vi "Begin.vi"(8 "error in":errorcluster) -> (0 "error out":errorcluster)   [LabVIEW 2015]
doc: "Called before other user functions, this VI is expected to open initial I/O refnums, load in file data, and do all program initialization. Notice that the <B>error out</B> terminal is simply used for data flow. Wiring it to other structures or subVIs ensures that this VI runs first."
uses:
  <vilib>/Rock Robotics/WPI/DriverStation/WPI_DriverStationRobotMode2.ctl
  <vilib>/Rock Robotics/WPI/Joystick/WPI_JoystickDeviceEnum.ctl
  <vilib>/Rock Robotics/SystemInterfaces/spilib/spi_bus.ctl
  <vilib>/Rock Robotics/WPI/SafetyOutput/WPI_SafetyOutputConfigMenu.ctl
  <vilib>/Rock Robotics/SystemInterfaces/DIO/FPGA_DIOPWMChannel.ctl
  <vilib>/Rock Robotics/SystemInterfaces/DIO/FPGA_DIOChannel.ctl
  <vilib>/Rock Robotics/WPI/Encoder/WPI_EncoderType.ctl
  <vilib>/Rock Robotics/WPI/CAN/TalonSRX/WPI_CANTalonSRX_APIControlMode.ctl
  Robot Global Data.vi
  <vilib>/Rock Robotics/Network Tables/NT Write String Array.vi
  <vilib>/Rock Robotics/WPI/Gyro/WPI_GyroXRS450_SPI_Open.vi
  GyroPlaceHolder.vi
  GyroLastValue.vi
  <vilib>/Rock Robotics/WPI/RobotDrive/WPI_RobotDriveOpen4MotorWithCANTalonSRX.vi
  <vilib>/Rock Robotics/WPI/MotorControl/WPI_MotorControlOpen TalonSRX.vi
  <vilib>/Rock Robotics/WPI/Counter/WPI_CounterDigitalInputToDigitalSource.vi
  <vilib>/Rock Robotics/WPI/MotorControl/WPI_MotorControlOpenCANTalonSRX.vi
  <vilib>/Rock Robotics/WPI/Switch/WPI_SwitchOpenLimit.vi
  <vilib>/Rock Robotics/WPI/Accelerometer/InternalAccelerometer/WPI_AccelerometerInternalOpen.vi
  <vilib>/Rock Robotics/SystemInterfaces/AI/FPGA_AIGyroChannel.ctl
  <vilib>/Rock Robotics/WPI/MotorControl/WPI_MotorControlOpen Talon.vi
  <vilib>/Rock Robotics/WPI/Gyro/WPI_GyroAnalogOpen.vi
  <vilib>/Rock Robotics/SystemInterfaces/i2clib/i2c_bus.ctl
  <vilib>/Rock Robotics/WPI/Accelerometer/ADXL345 Range.ctl
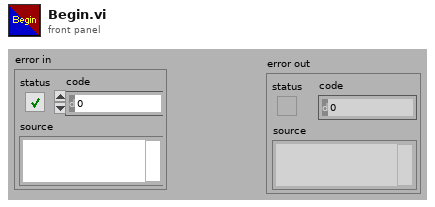
[diagram p1: front panel]
types:
  T1 = typedef "FPGA_DIOChannel.ctl" = enum8{"DIO 0", "DIO 1", "DIO 2", "DIO 3", "DIO 4", "DIO 5", "DIO 6", "DIO 7", "DIO 8", "DIO 9", "DIO MXP 0", "DIO MXP 1", "DIO MXP 2", "DIO MXP 3", "DIO MXP 4", "DIO MXP 5", "DIO MXP 6", "DIO MXP 7", "DIO MXP 8", "DIO MXP 9", "DIO MXP 10", "DIO MXP 11", "DIO MXP 12", "DIO MXP 13", "DIO MXP 14", "DIO MXP 15", "Invalid"}
  T2 = typedef "FPGA_DIOPWMChannel.ctl" = enum8{"PWM 0", "PWM 1", "PWM 2", "PWM 3", "PWM 4", "PWM 5", "PWM 6", "PWM 7", "PWM 8", "PWM 9", "PWM MXP 0", "PWM MXP 1", "PWM MXP 2", "PWM MXP 3", "PWM MXP 4", "PWM MXP 5", "PWM MXP 6", "PWM MXP 7", "PWM MXP 8", "PWM MXP 9", "Invalid"}
  T3 = typedef "WPI_EncoderType.ctl" = enum16{"1x", "2x", "4x"}
  T4 = typedef "WPI_CANTalonSRX_APIControlMode.ctl" = enum8{"Percent VBus", "Speed", "Position", "Slave", "Unchanged / Invalid", "Voltage Compensation", "Current", "Motion Profile"}
  T5 = typedef "WPI_JoystickDeviceEnum.ctl" = enum16{"USB 0", "USB 1", "USB 2", "USB 3", "USB 4", "USB 5"}
  T6 = typedef "WPI_SafetyOutputConfigMenu.ctl" = enum16{"Enable", "Disable"}
  T7 = typedef "spi_bus.ctl" = enum16{"SPI On-Board, CS0", "SPI On-Board, CS1", "SPI On-Board, CS2", "SPI On-Board, CS3", "SPI MXP", "Invalid"}
  T8 = typedef "WPI_DriverStationRobotMode2.ctl" = enum16{"Autonomous Disabled", "Autonomous Enabled", "Teleop Disabled", "Teleop Enabled", "Disconnected", "Finish", "Test Disabled", "Test Enabled", "Emergency Stopped"}
  T9 = typedef "FPGA_AIGyroChannel.ctl" = enum8{"AI 0", "AI 1", "Invalid"}
  T10 = typedef "WPI_AccelerometerDevRef.ctl" = cluster{"DevStatus":errorcluster, "Scaling":T11, "Analog Channels":T12, "I2C Bus":T14, "SPI Bus":T7, "Accel Range":T15, "ADXL Axes":T16, "Handle":i32, "Device Address":u8, "Accel Type":enum16{"Analog", "ADXL345 I2C", "ADXL345 SPI", "Internal", "ADXL362 SPI"}}
  T11 = typedef "WPI_AccelerometerScaling.ctl" = cluster{"Gain (VoltsPerG)":dbl, "Center Voltage":dbl}
  T12 = typedef "WPI_AccelerometerAnalogChannels.ctl" = cluster{"X-Axis":T13, "Y-Axis":T13, "Z-Axis":T13}
  T13 = typedef "FPGA_AIChannel.ctl" = enum8{"AI 0", "AI 1", "AI 2", "AI 3", "AI MXP 0", "AI MXP 1", "AI MXP 2", "AI MXP 3", "Invalid"}
  T14 = typedef "i2c_bus.ctl" = enum16{"I2C On-Board", "I2C MXP", "Invalid"}
  T15 = typedef "ADXL345 Range.ctl" = u8
  T16 = typedef "WPI_AccelerometerADXL345 Axes.ctl" = cluster{"X-Axis":bool, "Y-Axis":bool, "Z-Axis":bool}
  T17 = typedef "WPI_GyroDevRef.ctl" = cluster{"DevStatus":errorcluster, "Analog Channel":T13, "Offset":dbl, "Gain (VoltsPerDegree/Second)":dbl, "Gyro Type":enum16{"Analog", "XRS450"}, "Handle":i32, "SPI Bus":T7, "Device Found":bool, "Sample Rate":dbl, "Calibrate On Open":bool}
  T18 = typedef "WPI_CameraDevRef.ctl" = cluster{"Camera Address":string, "CameraStatus":errorcluster}
  T19 = typedef "WPI_DigitalInputDevRef.ctl" = cluster{"DevStatus":errorcluster, "DIO Channel":T1}
  T20 = typedef "FPGA_CounterEncoderSourceConvertionLVSourceType.ctl" = cluster{"DevStatus":errorcluster, "AnalogTriggerMode?":bool, "DigitalMode":cluster{"DIO Channel":T21}, "AnalogTriggerMode":cluster{"AnalogTriggerIndex":T22, "OutputType":T23}}
  T21 = typedef "FPGA_DIODigitalSourceChannel.ctl" = enum8{"DIO 0", "DIO 1", "DIO 2", "DIO 3", "DIO 4", "DIO 5", "DIO 6", "DIO 7", "DIO 8", "DIO 9", "DIO MXP 0", "DIO MXP 1", "DIO MXP 2", "DIO MXP 3", "DIO MXP 4", "DIO MXP 5", "DIO MXP 6", "DIO MXP 7", "DIO MXP 8", "DIO MXP 9", "DIO MXP 10", "DIO MXP 11", "DIO MXP 12", "DIO MXP 13", "DIO MXP 14", "DIO MXP 15", "Disabled"}
  T22 = typedef "FPGA_AnalogTriggerIndex.ctl" = enum8{"Trig 0", "Trig 1", "Trig 2", "Trig 3", "Trig 4", "Trig 5", "Trig 6", "Trig 7", "Invalid"}
  T23 = typedef "FPGA_AnalogTriggerOutType.ctl" = enum16{"InWindow", "TriggerState", "Rising", "Falling"}
  T24 = typedef "WPI_EncoderDevRef.ctl" = cluster{"DevStatus":errorcluster, "EncoderIndex":T25, "CounterIndex":T26, "DistancePerCount":dbl, "Decoding Type":T3}
  T25 = typedef "FPGA_EncoderIdx.ctl" = enum8{"Enc 0", "Enc 1", "Enc 2", "Enc 3", "Enc 4", "Enc 5", "Enc 6", "Enc 7", "Invalid"}
  T26 = typedef "FPGA_CounterCtrSystemIndex.ctl" = enum8{"Ctr 0", "Ctr 1", "Ctr 2", "Ctr 3", "Ctr 4", "Ctr 5", "Ctr 6", "Ctr 7", "Invalid"}
  T27 = typedef "WPI_JoystickDevRef.ctl" = cluster{"Device":T5}
  T28 = typedef "WPI_MotorControlDeviceRef.ctl" = cluster{"DeviceStatus":errorcluster, "Type":T29, "PWM":cluster{"PWM Channel":T2, "DeadBand":T30}, "CAN":cluster{"Device Number":u8, "Control Mode":T31, "Semaphore":T32, "Max Vout":dbl, "TalonSRX Control Mode":T4}, "Invert":bool}
  T29 = typedef "WPI_MotorControlType.ctl" = enum16{"PWM", "CAN", "CANTalonSRX"}
  T30 = typedef "WPI_PWMDeadband.ctl" = cluster{"Name":string, "maxPositivePwm":i32, "minPositivePwm":i32, "centerPwm":i32, "maxNegativePwm":i32, "minNegativePwm":i32, "angularRange":u16}
  T31 = typedef "WPI_CANJaguar_ControlMode.ctl" = enum8{"Percent VBus", "Current", "Speed", "Position", "Voltage"}
  T32 = typedef "Semaphore RefNum" = refnum<k1>
  T33 = typedef "WPI_RobotDriveDevRef.ctl" = cluster{"DevStatus":errorcluster, "Motors[]":T28[], "Square Inputs":bool, "Max Output":dbl}
  T34 = typedef "WPI_I2CDevRef.ctl" = cluster{"DevStatus":errorcluster, "Device Address":u8, "Handle":i32, "I2C Bus":T14}
  T35 = typedef "WPI_SwitchDevRef.ctl" = cluster{"DevStatus":errorcluster, "DIO Channel":T1, "CntIndex":T26, "Normally Closed":bool}
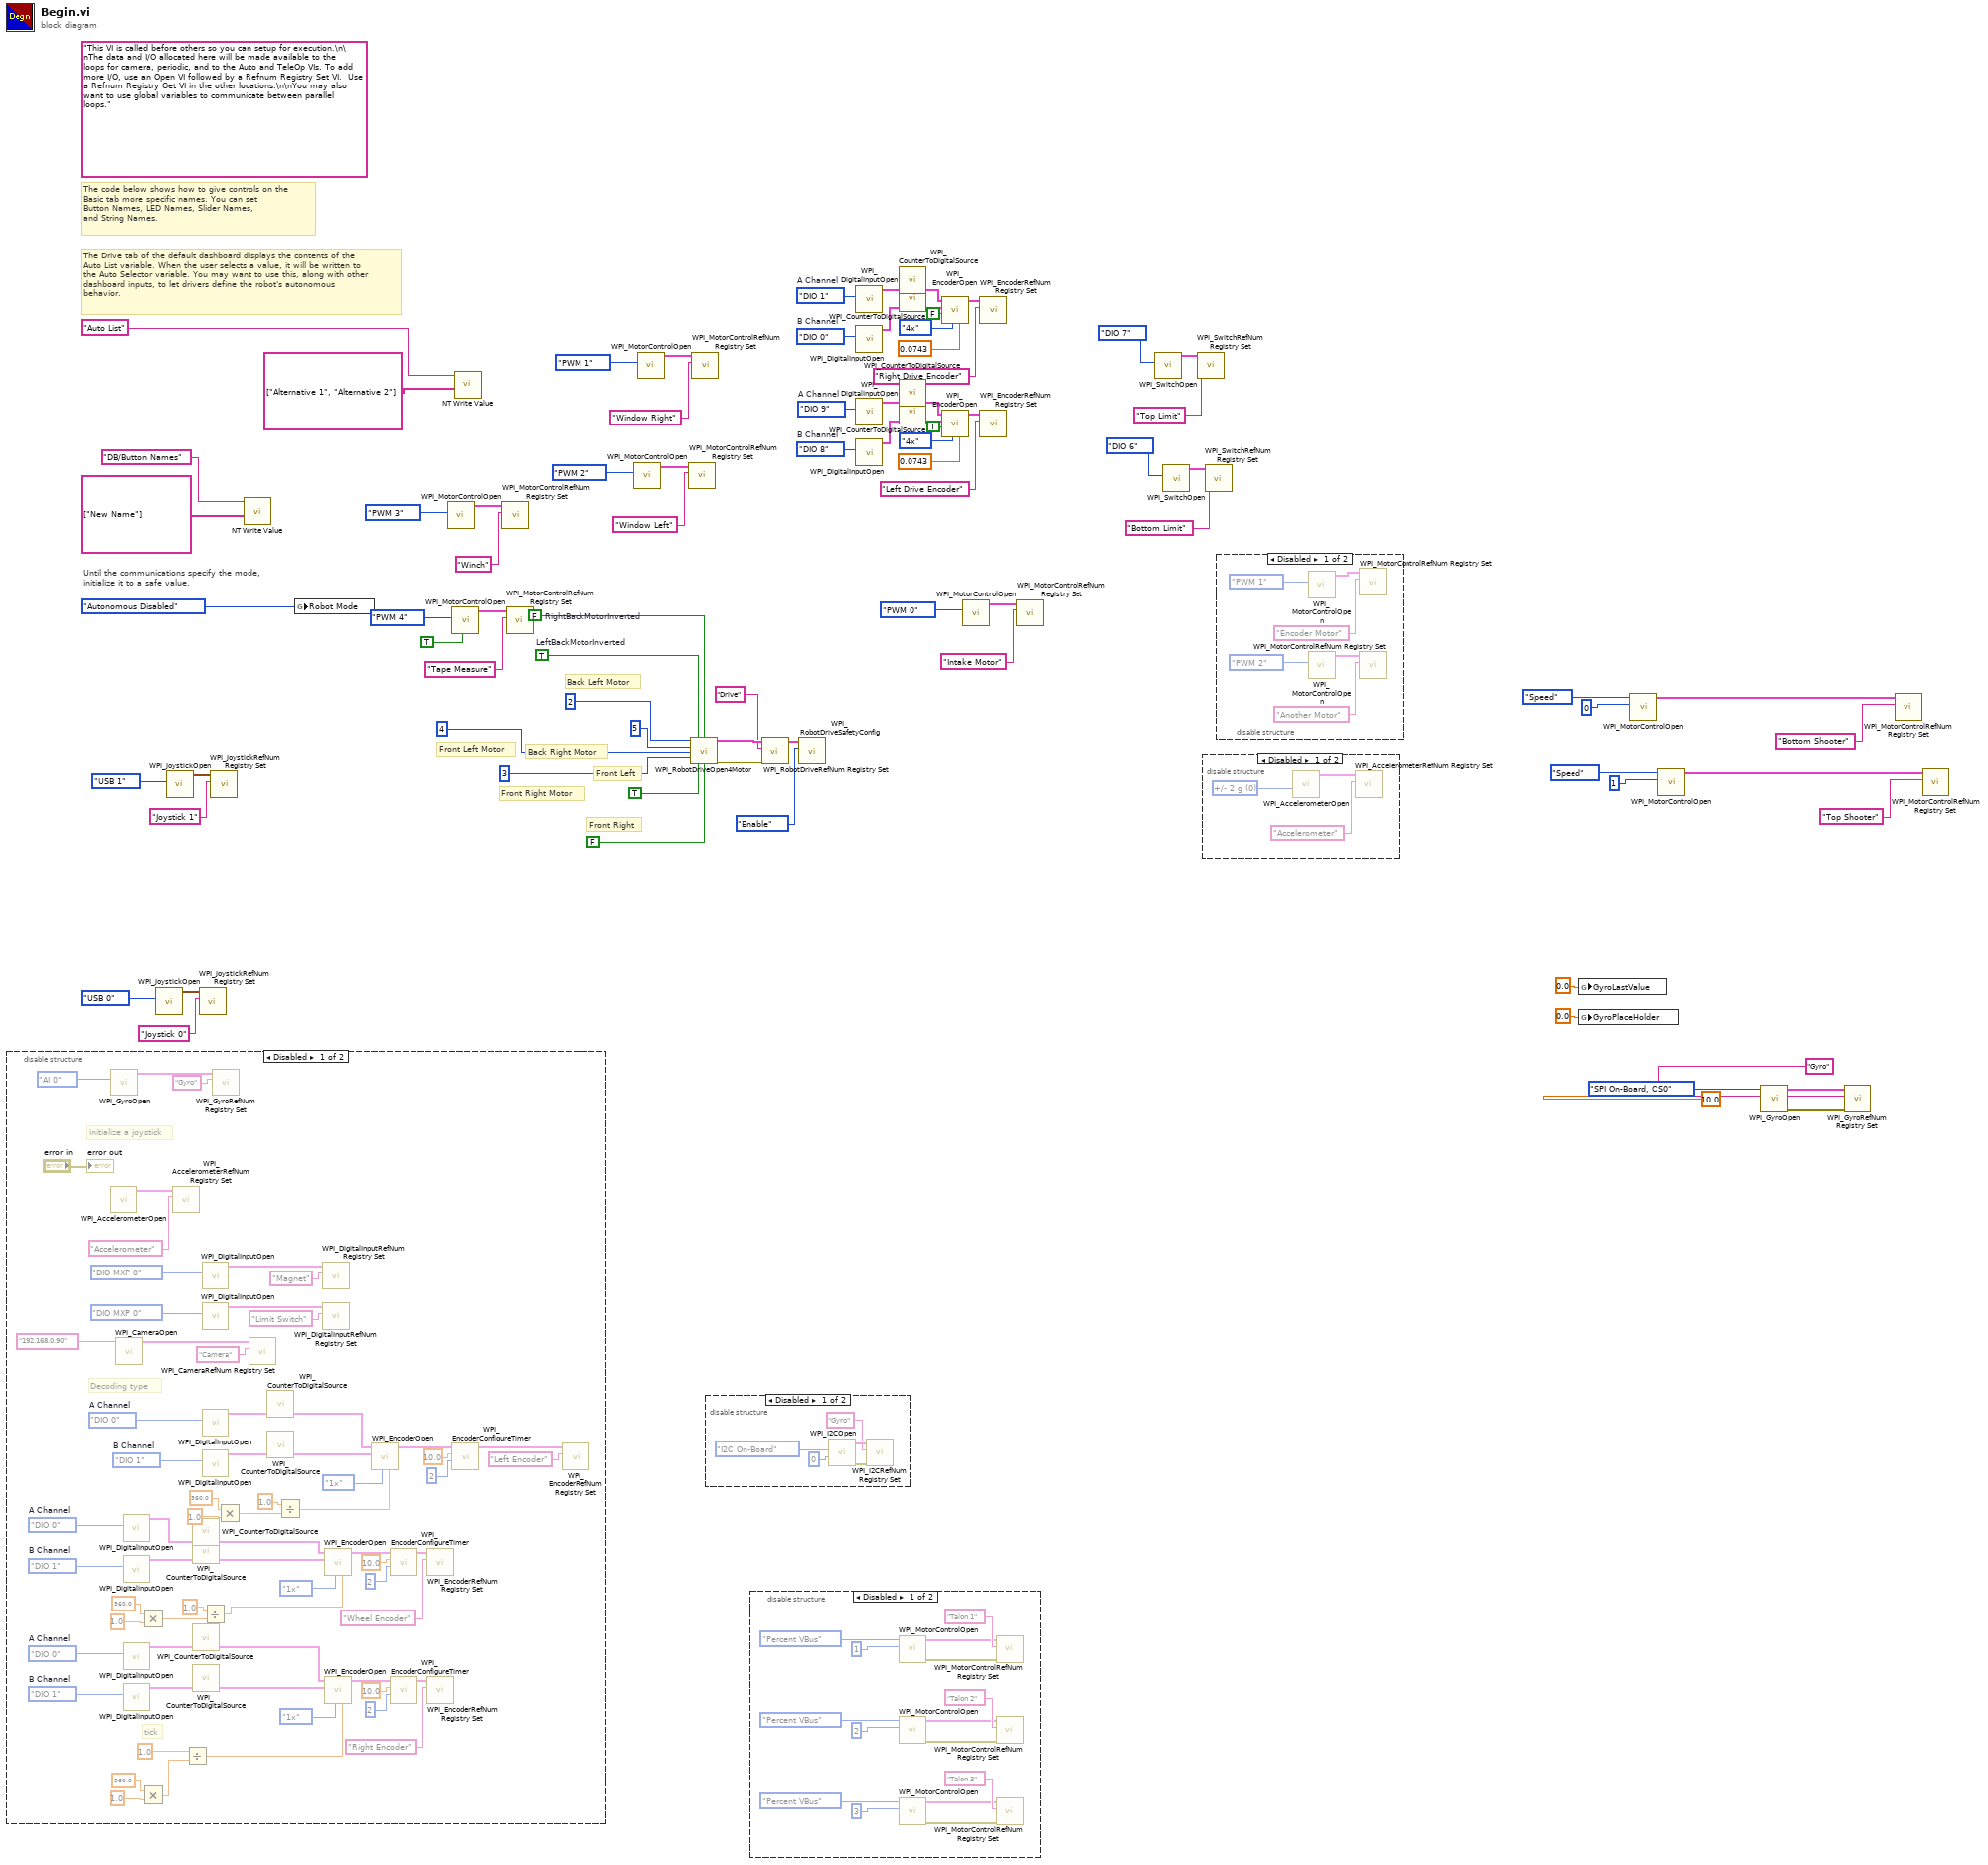
[diagram p0: block diagram]
diagram:
  w22 = FPGA_DIOChannel."DIO 8"  # B Channel
  w21 = FPGA_DIOChannel."DIO 9"  # A Channel
  w43 = FPGA_DIOChannel."DIO 0"  # B Channel
  w42 = FPGA_DIOChannel."DIO 1"  # A Channel
  w67 = TRUE  # LeftBackMotorInverted
  w68 = FALSE  # RightBackMotorInverted
  (unwired) "This VI is called before others so you can setup for execution.\n\nThe data and I/O allocated here will be made available to the loops for camera, periodic, and to the Auto and TeleOp VIs. To add more I/O, use an Open VI followed by a Refnum Registry Set VI.  Use a Refnum Registry Get VI in the other locations.\n\nYou may also want to use global variables to communicate between parallel loops."
  # "Front Right Motor"
  # "Front Left Motor"
  # "Back Left Motor"
  # "Back Right Motor"
  # "Front Right"
  # "Front Left"
  # "The Drive tab of the default dashboard displays the contents of the\nAuto List variable. When the user selects a value, it will be written to\nthe Auto Selector variable. You may want to use this, along with other\ndashboard inputs, to let drivers define the robot's autonomous\nbehavior."
  # "The code below shows how to give controls on the\nBasic tab more specific names. You can set\nButton Names, LED Names, Slider Names,\nand String Names."
  # "Until the communications specify the mode,\ninitialize it to a safe value."
  n1 = disable-structure shown="Disabled" {
    frame Disabled {
      w100 = FPGA_DIOChannel."DIO 1"  # B Channel
      w99 = FPGA_DIOChannel."DIO 0"  # A Channel
      w117 = FPGA_DIOChannel."DIO 1"  # B Channel
      w116 = FPGA_DIOChannel."DIO 0"  # A Channel
      w134 = FPGA_DIOChannel."DIO 1"  # B Channel
      w133 = FPGA_DIOChannel."DIO 0"  # A Channel
      # "tick"
      # "Decoding type"
      # "initialize a joystick"
      n2 = call-poly <vilib>:"WPI_AccelerometerOpen.vi"() -> ("AccelerometerDevRef"=w144:T10)  [unwired: 10 in, 1 out]
      n3 = call-poly <vilib>:"WPI_GyroOpen.vi"("Analog Channel"=FPGA_AIGyroChannel."AI 0") -> ("GyroDevRef"=w148:T17)  [unwired: 8 in, 2 out]
      n4 = call <vilib>:"WPI_CameraOpen.vi"("Camera Address"="192.168.0.90") -> ("CameraDevRef"=w147:T18)  [unwired: 9 in, 1 out]
      n5 = call <vilib>:"WPI_DigitalInputOpen.vi"("DIO Channel"=w133) -> ("DigitalInputDevRef"=w130:T19)  [unwired: 1 in, 9 out]
      n6 = call <vilib>:"WPI_DigitalInputOpen.vi"("DIO Channel"=w134) -> ("DigitalInputDevRef"=w131:T19)  [unwired: 1 in, 9 out]
      n7 = call <vilib>:"WPI_DigitalInputOpen.vi"("DIO Channel"=w116) -> ("DigitalInputDevRef"=w113:T19)  [unwired: 1 in, 9 out]
      n8 = call <vilib>:"WPI_DigitalInputOpen.vi"("DIO Channel"=w117) -> ("DigitalInputDevRef"=w114:T19)  [unwired: 1 in, 9 out]
      n9 = Multiply(x=360.0, y=1.0) -> (x*y=w120:dbl)
      n10 = Multiply(x=360.0, y=1.0) -> (x*y=w103:dbl)
      n11 = call <vilib>:"WPI_AccelerometerRefNum Registry Set.vi"("refnum name"="Accelerometer", "AccelerometerDevRef"=w144) -> ()  [unwired: 8 in, 2 out]
      n12 = Divide(x=1.0, y=w103) -> (x/y=w105:dbl)
      n13 = call-poly <vilib>:"WPI_CounterToDigitalSource.vi"("DigitalInputDevRef"=w130) -> ("Digital Source"=w129:T20)  [unwired: 6 out]
      n14 = call-poly <vilib>:"WPI_CounterToDigitalSource.vi"("DigitalInputDevRef"=w131) -> ("Digital Source"=w132:T20)  [unwired: 6 out]
      n15 = call-poly <vilib>:"WPI_CounterToDigitalSource.vi"("DigitalInputDevRef"=w113) -> ("Digital Source"=w112:T20)  [unwired: 6 out]
      n16 = call-poly <vilib>:"WPI_CounterToDigitalSource.vi"("DigitalInputDevRef"=w114) -> ("Digital Source"=w115:T20)  [unwired: 6 out]
      n17 = call <vilib>:"WPI_DigitalInputOpen.vi"("DIO Channel"=FPGA_DIOChannel."DIO MXP 0") -> ("DigitalInputDevRef"=w142:T19)  [unwired: 9 in, 1 out]
      n18 = call <vilib>:"WPI_DigitalInputOpen.vi"("DIO Channel"=FPGA_DIOChannel."DIO MXP 0") -> ("DigitalInputDevRef"=w137:T19)  [unwired: 9 in, 1 out]
      n19 = call <vilib>:"WPI_DigitalInputOpen.vi"("DIO Channel"=w99) -> ("DigitalInputDevRef"=w96:T19)  [unwired: 1 in, 9 out]
      n20 = call <vilib>:"WPI_DigitalInputOpen.vi"("DIO Channel"=w100) -> ("DigitalInputDevRef"=w97:T19)  [unwired: 1 in, 9 out]
      n21 = Divide(x=1.0, y=w120) -> (x/y=w122:dbl)
      n22 = call <vilib>:"WPI_GyroRefNum Registry Set.vi"("refnum name"="Gyro", "GyroDevRef"=w148) -> ()  [unwired: 8 in, 2 out]
      n23 = Multiply(x=360.0, y=1.0) -> (x*y=w86:dbl)
      n24 = call <vilib>:"WPI_CameraRefNum Registry Set.vi"("refnum name"="Camera", "CameraDevRef"=w147) -> ()  [unwired: 8 in, 2 out]
      n25 = call-poly <vilib>:"WPI_CounterToDigitalSource.vi"("DigitalInputDevRef"=w96) -> ("Digital Source"=w95:T20)  [unwired: 6 out]
      n26 = call-poly <vilib>:"WPI_CounterToDigitalSource.vi"("DigitalInputDevRef"=w97) -> ("Digital Source"=w98:T20)  [unwired: 6 out]
      n27 = Divide(x=1.0, y=w86) -> (x/y=w88:dbl)
      n28 = call <vilib>:"WPI_DigitalInputRefNum Registry Set.vi"("refnum name"="Magnet", "DigitalInputDevRef"=w142) -> ()  [unwired: 8 in, 2 out]
      n29 = call <vilib>:"WPI_DigitalInputRefNum Registry Set.vi"("refnum name"="Limit Switch", "DigitalInputDevRef"=w137) -> ()  [unwired: 8 in, 2 out]
      n30 = call <vilib>:"WPI_EncoderOpen.vi"("DistancePerCount"=w122, "Decoding Type"=WPI_EncoderType."1x", "BSource"=w132, "ASource"=w129) -> ("EncoderDevRef"=w125:T24)  [unwired: 4 in, 3 out]
      n31 = call <vilib>:"WPI_EncoderOpen.vi"("DistancePerCount"=w105, "Decoding Type"=WPI_EncoderType."1x", "BSource"=w115, "ASource"=w112) -> ("EncoderDevRef"=w108:T24)  [unwired: 4 in, 3 out]
      n32 = call <vilib>:"WPI_EncoderOpen.vi"("DistancePerCount"=w88, "Decoding Type"=WPI_EncoderType."1x", "BSource"=w98, "ASource"=w95) -> ("EncoderDevRef"=w91:T24)  [unwired: 4 in, 3 out]
      n33 = call <vilib>:"WPI_EncoderConfigureTimer.vi"("Number Samples to Average"=u8 2, "Minimum Rate"=10.0, "EncoderDevRef"=w125) -> ("EncoderDevRef"=w124:T24)  [unwired: 7 in, 1 out]
      n34 = call <vilib>:"WPI_EncoderConfigureTimer.vi"("Number Samples to Average"=u8 2, "Minimum Rate"=10.0, "EncoderDevRef"=w108) -> ("EncoderDevRef"=w107:T24)  [unwired: 7 in, 1 out]
      n35 = call <vilib>:"WPI_EncoderRefNum Registry Set.vi"("refnum name"="Wheel Encoder", "EncoderDevRef"=w124) -> ()  [unwired: 8 in, 2 out]
      n36 = call <vilib>:"WPI_EncoderRefNum Registry Set.vi"("refnum name"="Right Encoder", "EncoderDevRef"=w107) -> ()  [unwired: 8 in, 2 out]
      n37 = call <vilib>:"WPI_EncoderConfigureTimer.vi"("Number Samples to Average"=u8 2, "Minimum Rate"=10.0, "EncoderDevRef"=w91) -> ("EncoderDevRef"=w90:T24)  [unwired: 7 in, 1 out]
      n38 = call <vilib>:"WPI_EncoderRefNum Registry Set.vi"("refnum name"="Left Encoder", "EncoderDevRef"=w90) -> ()  [unwired: 8 in, 2 out]
      "error out" <- "error in"
    }
    frame Enabled {
    }
  }
  n39 = call <vilib>:"WPI_JoystickOpen.vi"("JoystickDevice"=WPI_JoystickDeviceEnum."USB 0") -> ("JoystickDevRef"=w81:T27)  [unwired: 10 in]
  n40 = call <vilib>:"WPI_JoystickOpen.vi"("JoystickDevice"=WPI_JoystickDeviceEnum."USB 1") -> ("JoystickDevRef"=w58:T27)  [unwired: 10 in]
  n41 = call <vilib>:"WPI_JoystickRefNum Registry Set.vi"("refnum name"="Joystick 0", "JoystickDevRef"=w81) -> ()  [unwired: 8 in, 2 out]
  n42 = call <vilib>:"WPI_JoystickRefNum Registry Set.vi"("refnum name"="Joystick 1", "JoystickDevRef"=w58) -> ()  [unwired: 8 in, 2 out]
  n43 = call-poly <vilib>:"NT Write Value.vi"("String Array"=string[] ["New Name"], "Name"="DB/Button Names") -> ()  [unwired: 9 in, 1 out]
  n44 = global write "Robot Global Data.vi" "Robot Mode"(WPI_DriverStationRobotMode2."Autonomous Disabled" ("Robot Mode")) -> ()
  n45 = call-poly <vilib>:"WPI_MotorControlOpen.vi"("PWM Channel"=FPGA_DIOPWMChannel."PWM 3") -> ("MotorControlDeviceRef"=w33:T28)  [unwired: 9 in, 1 out]
  n46 = call-poly <vilib>:"WPI_MotorControlOpen.vi"("Invert"=TRUE, "PWM Channel"=FPGA_DIOPWMChannel."PWM 4") -> ("MotorControlDeviceRef"=w10:T28)  [unwired: 8 in, 1 out]
  n47 = call-poly <vilib>:"NT Write Value.vi"("String Array"=string[] ["Alternative 1", "Alternative 2"], "Name"="Auto List") -> ()  [unwired: 9 in, 1 out]
  n48 = call <vilib>:"WPI_MotorControlRefNum Registry Set.vi"("refnum name"="Winch", "MotorControlDevRef"=w33) -> ()  [unwired: 8 in, 2 out]
  n49 = call <vilib>:"WPI_MotorControlRefNum Registry Set.vi"("refnum name"="Tape Measure", "MotorControlDevRef"=w10) -> ()  [unwired: 8 in, 2 out]
  n50 = call-poly <vilib>:"WPI_MotorControlOpen.vi"("PWM Channel"=FPGA_DIOPWMChannel."PWM 2") -> ("MotorControlDeviceRef"=w46:T28)  [unwired: 9 in, 1 out]
  n51 = call-poly <vilib>:"WPI_MotorControlOpen.vi"("PWM Channel"=FPGA_DIOPWMChannel."PWM 1") -> ("MotorControlDeviceRef"=w49:T28)  [unwired: 9 in, 1 out]
  n52 = call <vilib>:"WPI_MotorControlRefNum Registry Set.vi"("refnum name"="Window Left", "MotorControlDevRef"=w46) -> ()  [unwired: 8 in, 2 out]
  n53 = call-poly <vilib>:"WPI_RobotDriveOpen4Motor.vi"("Rear Left Motor"=u8 2, "Rear Left Motor Inverted"=w67, "Rear Right Motor Inverted"=w68, "Rear Right Motor"=u8 5, "Front Left Motor"=u8 4, "Front Right Motor"=u8 3, "Front Left Motor Inverted"=TRUE, "Front Right Motor Inverted"=FALSE) -> ("RobotDriveDevRef"=w66:T33, "error out"=w64:errorcluster)  [unwired: 6 in]
  n54 = call <vilib>:"WPI_MotorControlRefNum Registry Set.vi"("refnum name"="Window Right", "MotorControlDevRef"=w49) -> ()  [unwired: 8 in, 2 out]
  n55 = disable-structure shown="Disabled" {
    frame Disabled {
      n56 = call <vilib>:"WPI_I2COpen.vi"("Device Address"=u8 0, "I2C Bus"=i2c_bus."I2C On-Board") -> ("error out"=w153:errorcluster, "I2CDevRef"=w154:T34)  [unwired: 8 in]
      n57 = call <vilib>:"WPI_I2CRefNum Registry Set.vi"("error in (no error)"=w153, "refnum name"="Gyro", "I2CDevRef"=w154) -> ()  [unwired: 7 in, 2 out]
    }
    frame Enabled {
    }
  }
  n58 = disable-structure shown="Disabled" {
    frame Disabled {
      n59 = call-poly <vilib>:"WPI_MotorControlOpen.vi"("Device Number"=u8 1, "Control Mode"=WPI_CANTalonSRX_APIControlMode."Percent VBus") -> ("error out"=w169:errorcluster, "MotorControlDeviceRef"=w157:T28)  [unwired: 8 in]
      n60 = call-poly <vilib>:"WPI_MotorControlOpen.vi"("Device Number"=u8 2, "Control Mode"=WPI_CANTalonSRX_APIControlMode."Percent VBus") -> ("error out"=w165:errorcluster, "MotorControlDeviceRef"=w156:T28)  [unwired: 8 in]
      n61 = call-poly <vilib>:"WPI_MotorControlOpen.vi"("Device Number"=u8 3, "Control Mode"=WPI_CANTalonSRX_APIControlMode."Percent VBus") -> ("error out"=w161:errorcluster, "MotorControlDeviceRef"=w155:T28)  [unwired: 8 in]
      n62 = call <vilib>:"WPI_MotorControlRefNum Registry Set.vi"("error in (no error)"=w169, "refnum name"="Talon 1", "MotorControlDevRef"=w157) -> ()  [unwired: 7 in, 2 out]
      n63 = call <vilib>:"WPI_MotorControlRefNum Registry Set.vi"("error in (no error)"=w165, "refnum name"="Talon 2", "MotorControlDevRef"=w156) -> ()  [unwired: 7 in, 2 out]
      n64 = call <vilib>:"WPI_MotorControlRefNum Registry Set.vi"("error in (no error)"=w161, "refnum name"="Talon 3", "MotorControlDevRef"=w155) -> ()  [unwired: 7 in, 2 out]
    }
    frame Enabled {
    }
  }
  n65 = call <vilib>:"WPI_RobotDriveRefNum Registry Set.vi"("error in (no error)"=w64, "refnum name"="Drive", "RobotDriveDevRef"=w66) -> ("RobotDriveDevRef"=w63:T33)  [unwired: 1 in, 7 out]
  n66 = call <vilib>:"WPI_RobotDriveSafetyConfig.vi"("mode"=WPI_SafetyOutputConfigMenu."Enable", "RobotDriveDevRef"=w63) -> ()  [unwired: 8 in, 2 out]
  n67 = call <vilib>:"WPI_DigitalInputOpen.vi"("DIO Channel"=w42) -> ("DigitalInputDevRef"=w39:T19)  [unwired: 1 in, 9 out]
  n68 = call <vilib>:"WPI_DigitalInputOpen.vi"("DIO Channel"=w43) -> ("DigitalInputDevRef"=w40:T19)  [unwired: 1 in, 9 out]
  n69 = call <vilib>:"WPI_DigitalInputOpen.vi"("DIO Channel"=w21) -> ("DigitalInputDevRef"=w18:T19)  [unwired: 1 in, 9 out]
  n70 = call <vilib>:"WPI_DigitalInputOpen.vi"("DIO Channel"=w22) -> ("DigitalInputDevRef"=w19:T19)  [unwired: 1 in, 9 out]
  n71 = call-poly <vilib>:"WPI_CounterToDigitalSource.vi"("DigitalInputDevRef"=w39) -> ("Digital Source"=w38:T20)  [unwired: 6 out]
  n72 = call-poly <vilib>:"WPI_CounterToDigitalSource.vi"("DigitalInputDevRef"=w40) -> ("Digital Source"=w41:T20)  [unwired: 6 out]
  n73 = call-poly <vilib>:"WPI_CounterToDigitalSource.vi"("DigitalInputDevRef"=w18) -> ("Digital Source"=w17:T20)  [unwired: 6 out]
  n74 = call-poly <vilib>:"WPI_CounterToDigitalSource.vi"("DigitalInputDevRef"=w19) -> ("Digital Source"=w20:T20)  [unwired: 6 out]
  n75 = call <vilib>:"WPI_EncoderOpen.vi"("DistancePerCount"=0.0743, "Decoding Type"=WPI_EncoderType."4x", "Invert Direction (False)"=FALSE, "BSource"=w41, "ASource"=w38) -> ("EncoderDevRef"=w36:T24)  [unwired: 3 in, 3 out]
  n76 = call <vilib>:"WPI_EncoderOpen.vi"("DistancePerCount"=0.0743, "Decoding Type"=WPI_EncoderType."4x", "Invert Direction (False)"=TRUE, "BSource"=w20, "ASource"=w17) -> ("EncoderDevRef"=w15:T24)  [unwired: 3 in, 3 out]
  n77 = call-poly <vilib>:"WPI_MotorControlOpen.vi"("PWM Channel"=FPGA_DIOPWMChannel."PWM 0") -> ("MotorControlDeviceRef"=w52:T28)  [unwired: 9 in, 1 out]
  n78 = call <vilib>:"WPI_EncoderRefNum Registry Set.vi"("refnum name"="Right Drive Encoder", "EncoderDevRef"=w36) -> ()  [unwired: 8 in, 2 out]
  n79 = call <vilib>:"WPI_EncoderRefNum Registry Set.vi"("refnum name"="Left Drive Encoder", "EncoderDevRef"=w15) -> ()  [unwired: 8 in, 2 out]
  n80 = call <vilib>:"WPI_MotorControlRefNum Registry Set.vi"("refnum name"="Intake Motor", "MotorControlDevRef"=w52) -> ()  [unwired: 8 in, 2 out]
  n81 = call-poly <vilib>:"WPI_SwitchOpen.vi"("DIO Channel"=FPGA_DIOChannel."DIO 7") -> ("SwitchDevRef"=w4:T35)  [unwired: 9 in, 1 out]
  n82 = call-poly <vilib>:"WPI_SwitchOpen.vi"("DIO Channel"=FPGA_DIOChannel."DIO 6") -> ("SwitchDevRef"=w7:T35)  [unwired: 9 in, 1 out]
  n83 = call <vilib>:"WPI_SwitchRefNum Registry Set.vi"("refnum name"="Top Limit", "SwitchDevRef"=w4) -> ()  [unwired: 8 in, 2 out]
  n84 = disable-structure shown="Disabled" {
    frame Disabled {
      w171 = T15 0 items=["+/- 2 g", "+/- 4 g", "+/- 8 g", "+/- 16 g"] ("Accel Range")
      n85 = call-poly <vilib>:"WPI_AccelerometerOpen.vi"("Accel Range"=w171) -> ("AccelerometerDevRef"=w172:T10)  [unwired: 9 in, 1 out]
      n86 = call <vilib>:"WPI_AccelerometerRefNum Registry Set.vi"("refnum name"="Accelerometer", "AccelerometerDevRef"=w172) -> ()  [unwired: 8 in, 2 out]
    }
    frame Enabled {
    }
  }
  n87 = call <vilib>:"WPI_SwitchRefNum Registry Set.vi"("refnum name"="Bottom Limit", "SwitchDevRef"=w7) -> ()  [unwired: 8 in, 2 out]
  n88 = disable-structure shown="Disabled" {
    frame Disabled {
      n89 = call-poly <vilib>:"WPI_MotorControlOpen.vi"("PWM Channel"=FPGA_DIOPWMChannel."PWM 1") -> ("MotorControlDeviceRef"=w178:T28)  [unwired: 9 in, 1 out]
      n90 = call-poly <vilib>:"WPI_MotorControlOpen.vi"("PWM Channel"=FPGA_DIOPWMChannel."PWM 2") -> ("MotorControlDeviceRef"=w175:T28)  [unwired: 9 in, 1 out]
      n91 = call <vilib>:"WPI_MotorControlRefNum Registry Set.vi"("refnum name"="Encoder Motor", "MotorControlDevRef"=w178) -> ()  [unwired: 8 in, 2 out]
      n92 = call <vilib>:"WPI_MotorControlRefNum Registry Set.vi"("refnum name"="Another Motor", "MotorControlDevRef"=w175) -> ()  [unwired: 8 in, 2 out]
    }
    frame Enabled {
    }
  }
  n93 = global write "GyroLastValue.vi" "GyroLastValue"(0.0 ("GyroLastValue")) -> ()
  n94 = global write "GyroPlaceHolder.vi" "GyroPlaceHolder"(0.0 ("GyroPlaceHolder")) -> ()
  n95 = call-poly <vilib>:"WPI_MotorControlOpen.vi"("Device Number"=u8 0, "Control Mode"=WPI_CANTalonSRX_APIControlMode."Speed") -> ("MotorControlDeviceRef"=w27:T28)  [unwired: 8 in, 1 out]
  n96 = call-poly <vilib>:"WPI_MotorControlOpen.vi"("Device Number"=u8 1, "Control Mode"=WPI_CANTalonSRX_APIControlMode."Speed") -> ("MotorControlDeviceRef"=w23:T28)  [unwired: 8 in, 1 out]
  n97 = call-poly <vilib>:"WPI_GyroOpen.vi"("Sample Rate (ms)"=10.0, "SPI Bus"=spi_bus."SPI On-Board, CS0") -> ("error out"=w73:errorcluster, "GyroDevRef"=w74:T17)  [unwired: 8 in]
  n98 = call <vilib>:"WPI_GyroRefNum Registry Set.vi"("error in (no error)"=w73, "refnum name"="Gyro", "GyroDevRef"=w74) -> ()  [unwired: 7 in, 2 out]
  n99 = call <vilib>:"WPI_MotorControlRefNum Registry Set.vi"("refnum name"="Bottom Shooter", "MotorControlDevRef"=w27) -> ()  [unwired: 8 in, 2 out]
  n100 = call <vilib>:"WPI_MotorControlRefNum Registry Set.vi"("refnum name"="Top Shooter", "MotorControlDevRef"=w23) -> ()  [unwired: 8 in, 2 out]
